vi "Monero-Main.vi"   [LabVIEW 2017]
uses:
  <vilib>/rvi/DataTransferAndStorage/Container/XNode/niFpgaContainer.xnode
  <vilib>/rvi/interface/RandomDataEmulation/nirviRandomDataFpgaMultiElementTemplate.vi
  <vilib>/Platform/TimedLoop/XDataNode/XDataNode.xnode
  <vilib>/Platform/TimedLoop/XDataNode/nitl_modes.ctl
  <vilib>/Platform/TimedLoop/XDataNode/XDNodeRunTimeDep.lvlib
  <vilib>/Platform/TimedLoop/XDataNode/wakeup.ctl
  <vilib>/Platform/TimedLoop/XDataNode/timing_clust.ctl
  Monero-FPGA-3/monero-3-data.ctl
  Monero-FPGA-3/Monero-FPGA-3.lvlib
  Monero-FPGA-3/monero-3-control.ctl
types:
  T1 = typedef "Monero-FPGA-3.lvlib/monero-3-control.ctl" = cluster{"data position-send-recv":i32, "Read FIFO?":bool, "Processing?":bool, "current iteration":u32, "Write FIFO?":bool, "Output Valid?":bool}
  T2 = typedef "Monero-FPGA-3.lvlib/monero-3-data.ctl" = cluster{"a0":u64, "a1":u64, "b0":u64, "b1":u64, "state-262143":u64[]}
  T3 = typedef "XDNodeRunTimeDep.lvlib/timing_clust.ctl" = cluster{"Expected End [f-1]":u64, "Actual End [f-1]":u64, "Finished Late? [f-1]":bool, "Expected End [i-1]":u64, "Actual End [i-1]":u64, "Finished Late? [i-1]":bool, "Expected Start [i]":u64, "Actual Start [i]":u64, "Expected Start [f]":u64, "Actual Start [f]":u64, "Source Name":string, "Structure Name":string, "Period":i64, "Deadline":i64, "Offset":i64, "Start":i64, "Priority":i32, "Timeout":i32, "Mode":T4, "Wakeup Reason":T5, "Error":errorcluster, "Source Type":string, "Secondary Source Type":string, "Global End Time":u64, "Global Start Time":u64, "Frame Duration":u64, "Iteration Duration":u64, "Assigned CPU":i32, "I/O Scan Engine Mode":u32}
  T4 = typedef "XDNodeRunTimeDep.lvlib/nitl_modes.ctl" = enum32{"No Change", "Process missed periods, maintain original phase", "Discard missed periods, maintain original phase", "Process missed periods, ignore original phase", "Discard missed periods, ignore original phase"}
  T5 = typedef "XDNodeRunTimeDep.lvlib/wakeup.ctl" = enum32{"Normal", "Aborted", "Asynchronous wakeup", "Timing source error", "Timed loop error", "Timeout"}
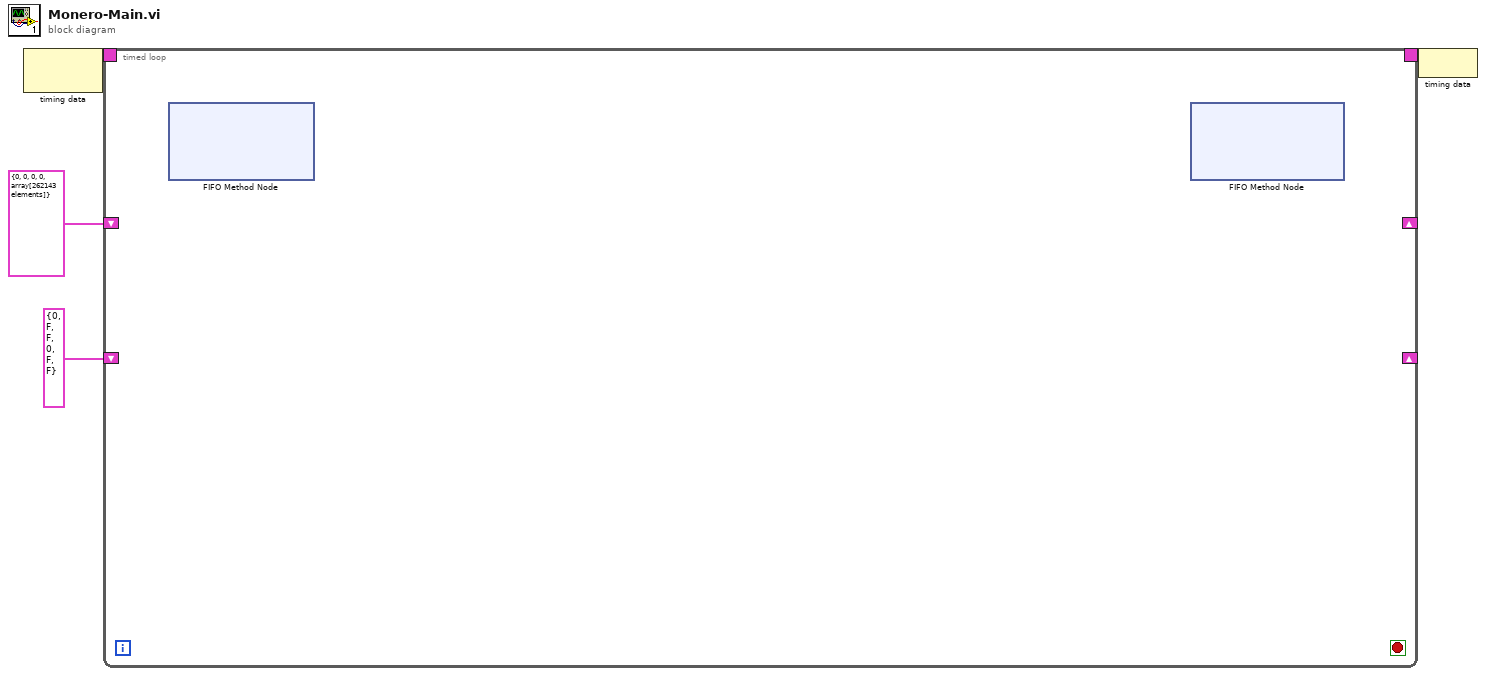
[diagram p0: block diagram]
diagram:
  n1 = node-c288() -> (w4:T3)  [unwired: 1 in]
  n2 = timed-loop {
    timing: w4 -> [_]
    timing-out: [_] -> w3
    shift-right: _ -> [_]
    shift-left: T2 {"a0"=0, "a1"=0, "b0"=0, "b1"=0, "state-262143"=array[262143 elements]} ("Monero-3") -> [_]
    shift-right: _ -> [_]
    shift-left: T1 {"data position-send-recv"=0, "Read FIFO?"=FALSE, "Processing?"=FALSE, "current iteration"=0, "Write FIFO?"=FALSE, "Output Valid?"=FALSE} ("monero-3-control") -> [_]
    stop <- _ stop-if-true
    n3 = xnode ("FIFO Method Node")() -> ()  [unwired: 2 in, 3 out]
    n4 = xnode ("FIFO Method Node")() -> ()  [unwired: 3 in, 2 out]
  }
  n5 = node-c288(w3) -> ()
